vi "Read Field XY Scalars.vi"(4 "YLinkData":T1, 6 "XLinkData":T1, 8 "Error In":errorcluster, 9 "YLink":T2, 10 "XLink":T2, 11 "WorkspaceManager":T3) -> (0 "Error Out":errorcluster, 1 "Values":cluster{"Values[0]":dbl, "Values[1]":dbl}, 2 "Changed?":bool)   [LabVIEW 2011]
uses:
  Controls/ECUMC Item.ctl
  Controls/LinkData.ctl
  <vilib>/NI Veristand/Execution/Workspace/WorkspaceAPI.ctl
  NationalInstruments.VeriStand.ClientAPI
  Check Link for Char or Meas.vi
  Tables/last part of path.vi
  <vilib>/ECUMC/NIVS/Get Meas Data.vi
  <vilib>/ECUMC/NIVS/Support Files.llb/Get Single Meas Data (TCP).vi
  <vilib>/ECUMC/NIVS/Get Char Data.vi
  <vilib>/ECUMC/NIVS/Support Files.llb/Get Single Char Data (TCP).vi
  <vilib>/NI Veristand/Execution/Workspace/NI VeriStand - Get Channel Value.vi
  <vilib>/NI Veristand/Execution/Workspace/NI VeriStand - Get Single Channel Value.vi
  <vilib>/NI Veristand/Execution/Workspace/NI_VS Workspace ExecutionAPI.lvlib
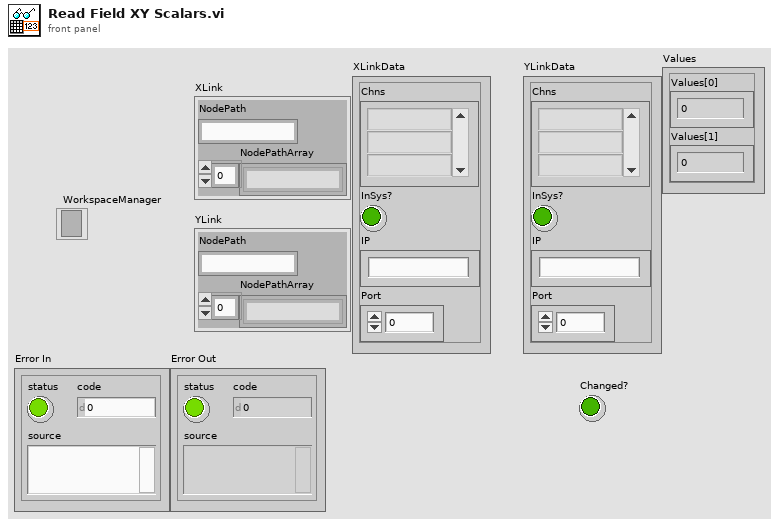
[diagram p1: front panel]
types:
  T1 = typedef "LinkData.ctl" = cluster{"Chns":string[], "InSys?":bool, "IP":string, "Port":u16}
  T2 = typedef "ECUMC Item.ctl" = cluster{"NodePath":string, "NodePathArray":string[]}
  T3 = typedef "NI_VS Workspace ExecutionAPI.lvlib/WorkspaceAPI.ctl" = refnum<k24>
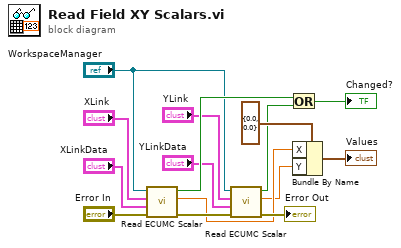
[diagram p0: block diagram]
diagram:
  n1 = call "Read ECUMC Scalar.vi"("Error In"="Error In", "LinkData"="XLinkData", "Link"="XLink", "WorkspaceManager"="WorkspaceManager") -> ("Error Out"=w14:errorcluster, "Value"=w8:dbl, "Changed?"=w7:bool)  [unwired: 5 in]
  n2 = call "Read ECUMC Scalar.vi"("Error In"=w14, "LinkData"="YLinkData", "Link"="YLink", "WorkspaceManager"="WorkspaceManager") -> ("Error Out"=→"Error Out":errorcluster, "Value"=w1:dbl, "Changed?"=w6:bool)  [unwired: 5 in]
  n3 = Or(x=w7, y=w6) -> (x .or. y?=→"Changed?":bool)
  n4 = Bundle By Name(cluster=cluster{"X":dbl, "Y":dbl} {"X"=0.0, "Y"=0.0} ("Values"), "X"=w8, "Y"=w1) -> (→"Values":cluster{"X":dbl, "Y":dbl})
